vi "runtest format Datasheet Printing Query.vi"(7 "Template (\"\")":string, 8 "Test Type (\"\")":string, 9 "Run (\"\")":string, 10 "Serial Number (\"\")":string, 11 "Model Number (\"\")":string) -> (3 "Datasheet Query":string)   [LabVIEW 2011]
uses:
  <vilib>/addons/internet/utils/strutil.llb/Case Matching.ctl
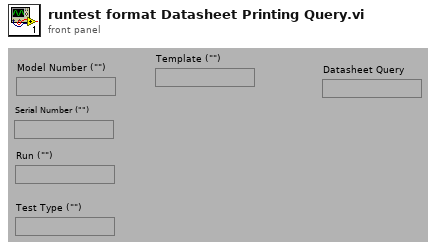
[diagram p1: front panel]
types:
  T1 = typedef "Case Matching.ctl" = enum16{"a != A", "a == A", "system"}
  T2 = typedef "Keyed Array.ctl" = cluster{"keys":string[], "values":string[]}
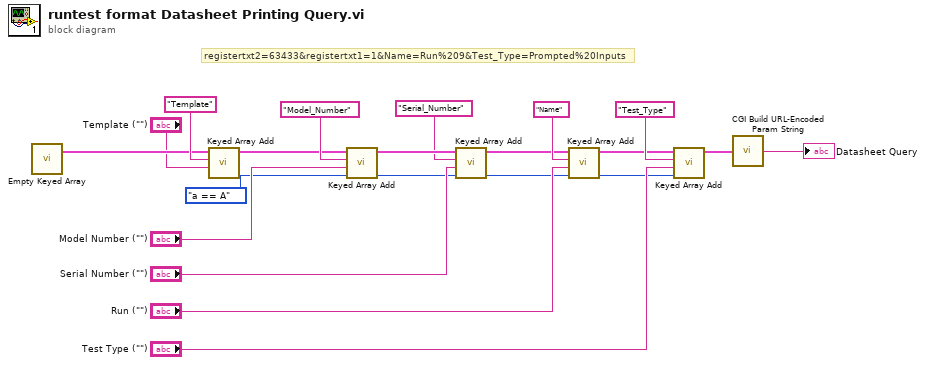
[diagram p0: block diagram]
diagram:
  w4 = Case_Matching."a == A" ("case matching (sensitive)")
  # "registertxt2=63433&registertxt1=1&Name=Run%209&Test_Type=Prompted%20Inputs"
  n1 = call "Empty Keyed Array.vi"() -> ("empty keyed array"=w5:T2)  [unwired: 3 out]
  n2 = call <vilib>:"Keyed Array Add.vi"("case matching (sensitive)"=w4, "value"="Template (\"\")", "key"="Template", "array in"=w5) -> ("array out"=w6:T2)  [unwired: 3 out]
  n3 = call <vilib>:"Keyed Array Add.vi"("case matching (sensitive)"=w4, "value"="Model Number (\"\")", "key"="Model_Number", "array in"=w6) -> ("array out"=w16:T2)  [unwired: 3 out]
  n4 = call <vilib>:"Keyed Array Add.vi"("case matching (sensitive)"=w4, "value"="Serial Number (\"\")", "key"="Serial_Number", "array in"=w16) -> ("array out"=w12:T2)  [unwired: 3 out]
  n5 = call <vilib>:"Keyed Array Add.vi"("case matching (sensitive)"=w4, "value"="Run (\"\")", "key"="Name", "array in"=w12) -> ("array out"=w9:T2)  [unwired: 3 out]
  n6 = call <vilib>:"Keyed Array Add.vi"("case matching (sensitive)"=w4, "value"="Test Type (\"\")", "key"="Test_Type", "array in"=w9) -> ("array out"=w2:T2)  [unwired: 3 out]
  n7 = call <vilib>:"CGI Build URL-Encoded Param String.vi"("params"=w2) -> ("url-encoded param string"=→"Datasheet Query":string)
